vi "Write and Read Multiple Registers.vi"(4 "read count":u16, 6 "read starting address":u16, 8 "error in":errorcluster, 9 "write values":u16[](array[numeric]), 10 "write starting address":u16, 11 "device data model in":refnum<class "Device Data Model.lvclass">) -> (0 "error out":errorcluster, 1 "read values":u16[](array[numeric]), 3 "device data model out":refnum<class "Device Data Model.lvclass">)   [LabVIEW 2012, in "Device Data Model.lvclass"]
doc: "Writes and reads the values of multiple register values in series. The <b>write values</b> are inserted starting at <b>write starting address</b> and the returned <b>read values</b> consists of <b>read count</b> holding registers starting at <b>read starting address</b>."
uses:
  Device Data Model.lvclass
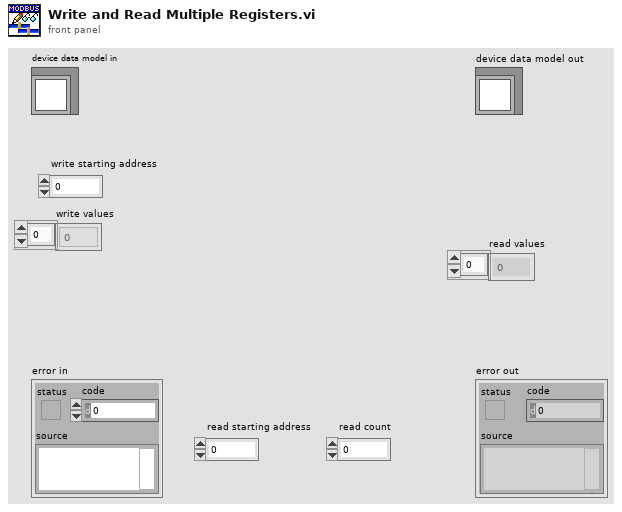
[diagram p1: front panel]
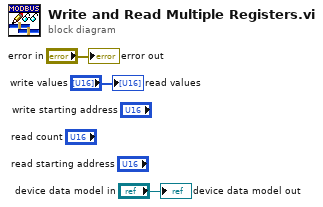
[diagram p0: block diagram]
diagram:
  "error out" <- "error in"
  "device data model out" <- "device data model in"
  "read values" <- "write values"
